vi "Actor Core.vi"(8 "error in":errorcluster, 11 "userInfoManage in":refnum<class "UserInfoManageUI.lvclass">) -> (0 "error out":errorcluster, 3 "Actor out":refnum<class "Actor.lvclass">)   [LabVIEW 2015, in "ActorManagement.lvlib" / "UserInfoManageUI.lvclass"]
doc: "(<B>Filename</B>: Actor Framework.lvlib:Actor.lvclass:Actor Core.vi)\n\nReceives messages to the actor, reacts to them, and initiates any error handling that may shut the actor down.\n\nDescendant classes may override this VI to append parallel tasks for the actor to complete while it handles messages. Overrides use the Call Parent Method node."
uses:
  UserInfoManageUI.lvclass
  <vilib>/ActorFramework/Actor/Actor.lvclass
  typedef/Member Basic Info(UI).ctl
  UserManagement/User/typedef/SchoolOfUser.ctl
  UserManagement/User/typedef/GradeOfUser.ctl
  UserManagement/User/typedef/GroupOfUser.ctl
  typedef/Member Search Condition(UI).ctl
  <vilib>/ActorFramework/Actor/Actor.lvclass/Actor.ctl
  <vilib>/ActorFramework/Message Enqueuer/Message Enqueuer.lvclass/Message Enqueuer.ctl
  Messages/Add Member to Database_Msg/Add Member to Database_Msg.lvclass/Add Member to Database_Msg.ctl
  <vilib>/ActorFramework/Stop Msg/Stop Msg.lvclass/Stop Msg.ctl
  <vilib>/ActorFramework/Message Enqueuer/Init from Existing Queue.vi
  <vilib>/ActorFramework/Message Enqueuer/Enqueue.vi
  <vilib>/ActorFramework/Message Enqueuer/Enqueue Critical.vi
  <vilib>/ActorFramework/Message Priority Queue/Priority Enqueue.vi
  PluginWithDatabase/PluginWithDatabase.lvclass
  <vilib>/ActorFramework/Message Enqueuer/Message Enqueuer.lvclass
  Messages/Add Member to Database_Msg/Add Member to Database_Msg.lvclass
  <vilib>/ActorFramework/Stop Msg/Stop Msg.lvclass
  UserManagement/UserBasicInfo/UserBasicInfo.lvclass
  UserManagement/User/User.lvclass
panel:
  in  "Tab Control":enum32{"添加队员信息", "查看队员信息"}(tab)
  in  "Member Basic Info":T1
  in  "Register":bool
  in  "Search":bool
  out "Table Control":string[][](table)
  in  "searchContent":T5
  in  "stop(test)":bool
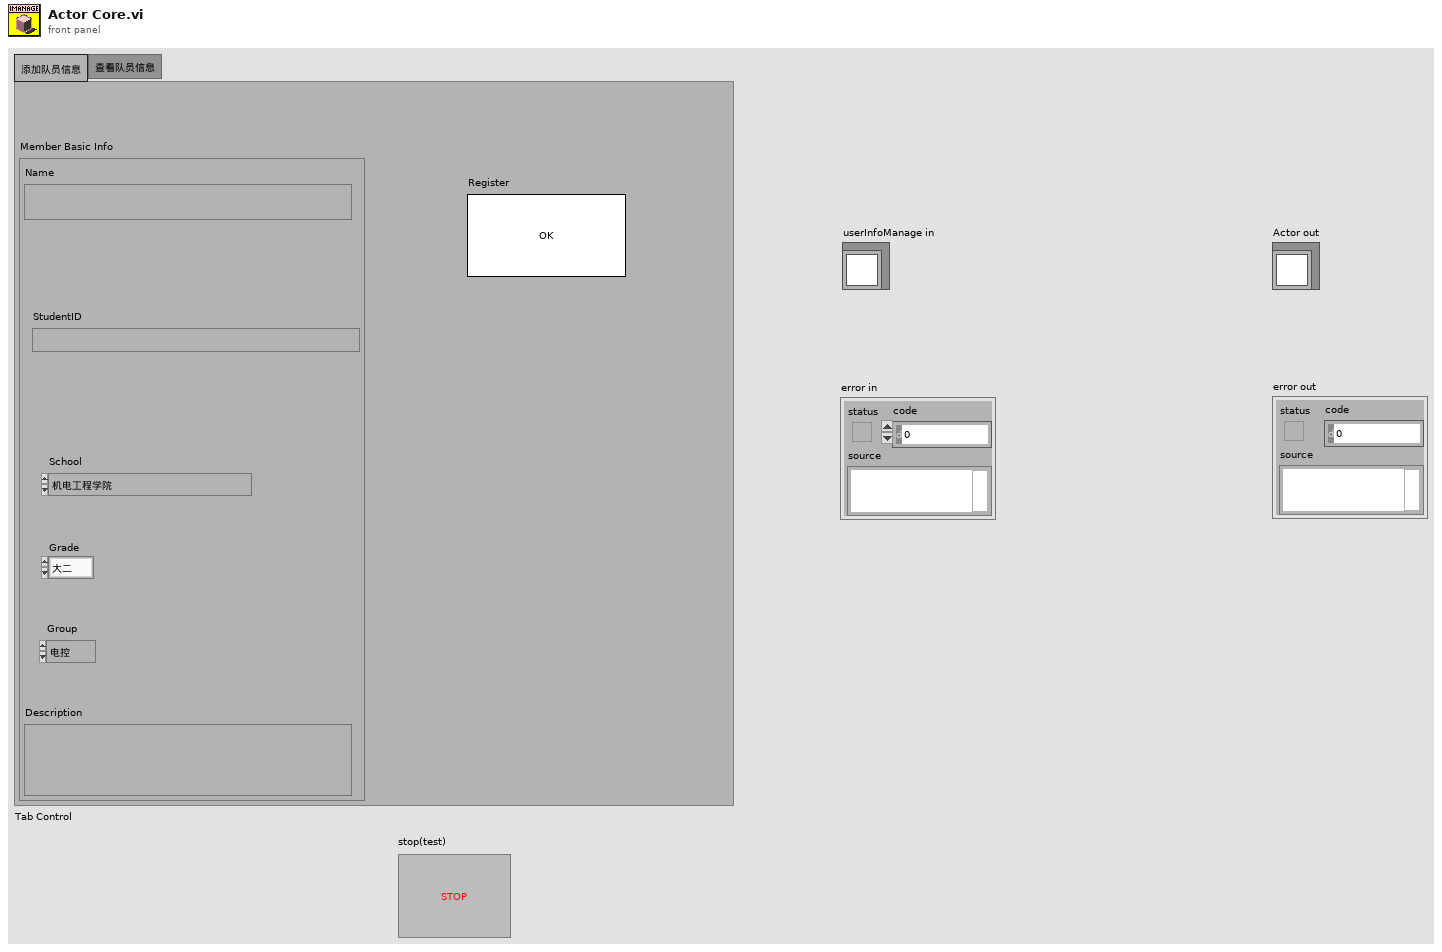
[diagram p1: front panel]
types:
  T1 = typedef "UserManagement.lvlib/UserBasicInfo.lvclass/Member Basic Info(UI).ctl" = cluster{"Name":string, "StudentID":string, "Description":string, "School":T2, "Grade":T3, "Group":T4}
  T2 = typedef "UserManagement.lvlib/User.lvclass/SchoolOfUser.ctl" = enum8{"机电工程学院", "电气工程学院", "航天学院", "能源学院", "理学院", "英才学院"}
  T3 = typedef "UserManagement.lvlib/User.lvclass/GradeOfUser.ctl" = enum16{"大二", "大三", "大四", "研一"}
  T4 = typedef "UserManagement.lvlib/User.lvclass/GroupOfUser.ctl" = enum16{"电控", "机械", "视觉"}
  T5 = typedef "UserManagement.lvlib/UserBasicInfo.lvclass/Member Search Condition(UI).ctl" = cluster{"学号":string, "姓名":string, "学院":enum16{"全体", "机电工程学院", "电气工程学院", "航天学院", "能源学院", "理学院", "英才学院"}, "年级":enum16{"全体", "大二", "大三", "大四", "研一"}, "组别":enum16{"全体", "电控", "机械", "视觉"}}
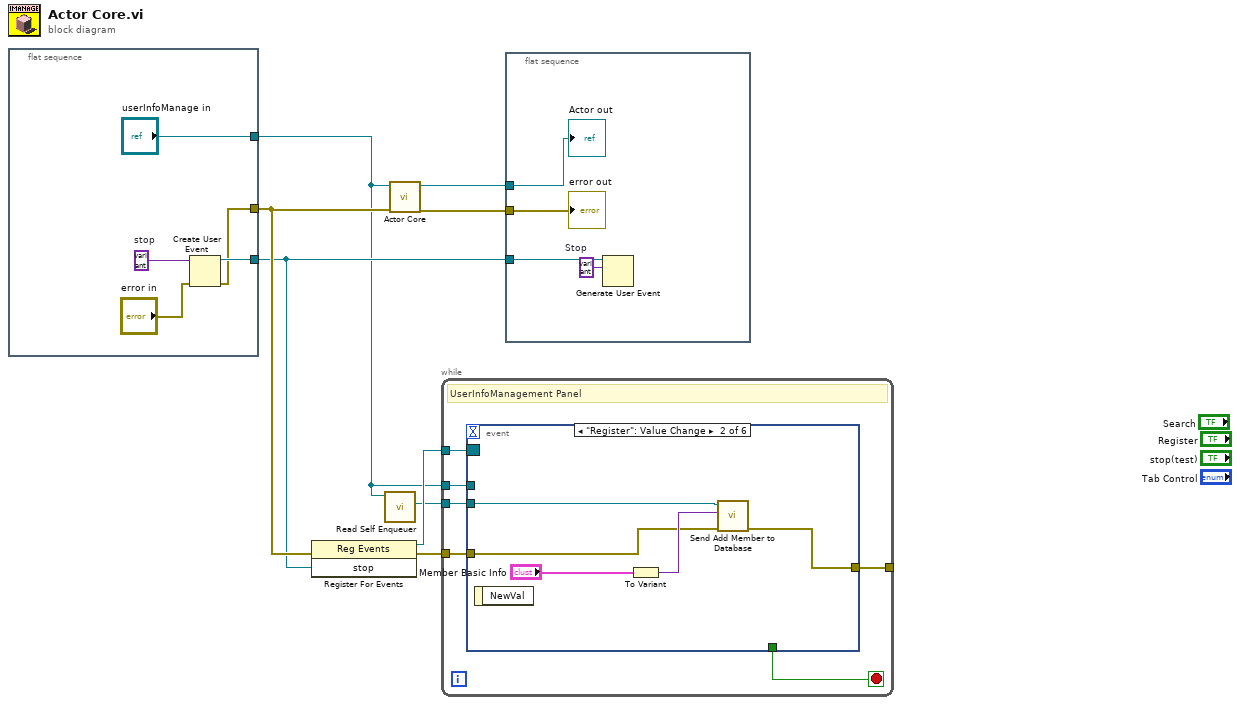
[diagram p0: block diagram]
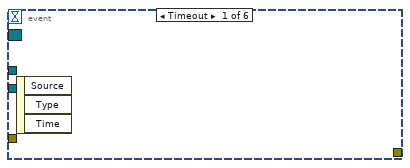
[diagram p2: hidden frame]
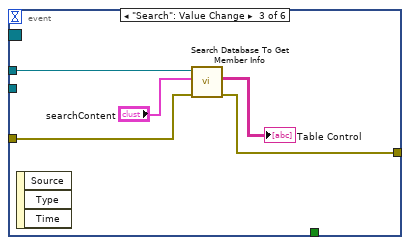
[diagram p3: hidden frame]
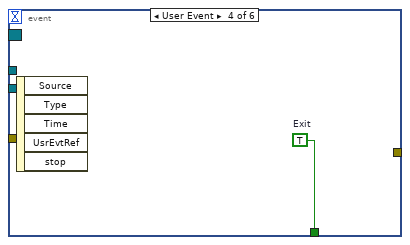
[diagram p4: hidden frame]
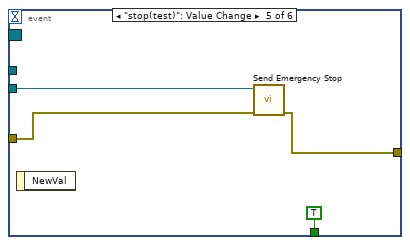
[diagram p5: hidden frame]
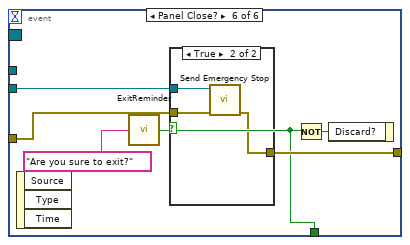
[diagram p6: hidden frame]
diagram:
  n1 = flat-sequence {
    tunnel: ["userInfoManage in"] -> w2
    tunnel: [w9] -> w6
    tunnel: [w11] -> w5
    frame #0 {
      w12 = variant  # stop
      n2 = Create User Event(user event datatype=w12, error in="error in") -> (user event=w11:refnum<user-event>, error out=w9:errorcluster)
    }
  }
  n3 = register-events(error in=w6, w5) -> (reference out=w3:refnum<event-registration>, error out=w4:errorcluster)  [unwired: 1 in]
  n4 = call <vilib>:"Read Self Enqueuer.vi"("Actor"=w2) -> ("Self Enqueuer"=w1:refnum<class "Message Enqueuer.lvclass">)  [unwired: 10 in]
  n5 = call-parent "Actor Core.vi"("error in"=w6, "Actor in"=w2) -> ("error out"=w8:errorcluster, "Actor out"=w7:refnum<class "Actor.lvclass">)  [unwired: 8 in]
  n6 = while {
    tunnel: w2 -> [w19]
    tunnel: w4 -> [w18]
    tunnel: w3 -> [w17]
    tunnel: w1 -> [w15]
    tunnel: [w14] -> _
    stop <- w16 stop-if-true
    # "UserInfoManagement Panel"
    n7 = event shown="[1] \"Register\": Value Change" {
      selector: w17 -> [_ _ _ _ _ _]
      dyn-events: _ -> [_ _ _ _ _ _]
      timeout: _ -> [_ _ _ _ _ _]
      tunnel: w19 -> [_ _ w29 _ _ _]
      tunnel: w18 -> [_ w21 w27 _ w33 w39]
      tunnel: [_ _ _ w30 TRUE ("Exit") w36] -> w16
      tunnel: w15 -> [_ w23 _ _ w34 w40]
      tunnel: [_ w20 w25 _ w32 w38] -> w14
      event Timeout {
        n8 = event-data() -> ()  [unwired: 1 in, 3 out]
      }
      event "Register": Value Change {
        n9 = event-data() -> ()  [unwired: 1 in, 1 out]
        n10 = To Variant(anything="Member Basic Info") -> (Variant=w22:variant)
        n11 = call "Send Add Member to Database.vi"("error in (no error)"=w21, "UI data"=w22, "Message Enqueuer"=w23) -> ("error out"=w20:errorcluster)  [unwired: 7 in, 1 out]
      }
      event "Search": Value Change {
        n12 = event-data() -> ()  [unwired: 1 in, 3 out]
        n13 = call "Search Database To Get Member Info.vi"("error in (no error)"=w27, "searchContent"="searchContent", "userInfoManage in"=w29) -> ("error out"=w25:errorcluster, "Result"=→"Table Control":string[][])  [unwired: 6 in, 1 out]
      }
      event User Event {
        w30 = TRUE  # Exit
        n14 = event-data() -> ()  [unwired: 1 in, 5 out]
      }
      event "stop(test)": Value Change {
        n15 = event-data() -> ()  [unwired: 1 in, 1 out]
        n16 = call <vilib>:"Send Emergency Stop.vi"("error in (no error)"=w33, "Message Enqueuer"=w34) -> ("error out"=w32:errorcluster)  [unwired: 9 in]
      }
      event Panel Close? {
        n17 = event-data() -> ()  [unwired: 1 in, 3 out]
        n18 = call "ExitReminder.vi"("message"="Are you sure to exit?") -> ("Exit"=w36:bool)
        n19 = case shown="True" w36 {
          tunnel: w40 -> [_ w44]
          tunnel: w39 -> [w41 w43]
          tunnel: [w41 w42] -> w38
          frame False {
          }
          frame True {
            n20 = call <vilib>:"Send Emergency Stop.vi"("error in (no error)"=w43, "Message Enqueuer"=w44) -> ("error out"=w42:errorcluster)  [unwired: 9 in]
          }
        }
        n21 = Not(x=w36) -> (.not. x?=w37:bool)
        n22 = event-data("Discard?"=w37) -> ()  [unwired: 1 in, 1 out]
      }
    }
  }
  n23 = flat-sequence {
    tunnel: w8 -> [w48]
    tunnel: w7 -> [w47]
    tunnel: w5 -> [w46]
    frame #0 {
      w45 = variant  # Stop
      n24 = Generate User Event(user event=w46, event data cluster=w45) -> ()  [unwired: 2 in, 2 out]
      "error out" <- w48
      "Actor out" <- w47
    }
  }
